vi "Create Analog Waveform.vi"(8 "error in (no error)":errorcluster, 9 "Type (0: awfSine)":i32(ring) items=["awfSine", "awfLoDistSine", "awfPhasedSine", "awfNoise", "awfUSASI", "awfSquare", "awfRamp", "awfArb", "awfChirp", "awfMultiTone", "awfIMD", "awfSyncBurstSine", "awfDC", "awfPolarity", "awfMLS", "awfLogSine"], 10 "Channel (0: A)":i32(ring) items=["A", "B"], 11 "VISA resource name":refnum<visa-resource-name>) -> (0 "error out":errorcluster, 2 "Waveform Channel ID":i32, 3 "VISA resource name out":refnum<visa-resource-name>)   [LabVIEW 2014, in "Stanford Research SR1.lvlib"]
doc: "Adds a waveform of the specified type to the generator channel and returns the ID of the newly created waveform."
uses:
  Stanford Research SR1.lvlib
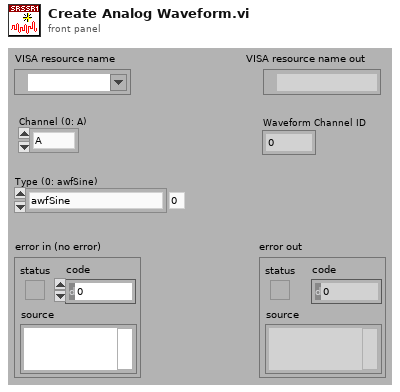
[diagram p1: front panel]
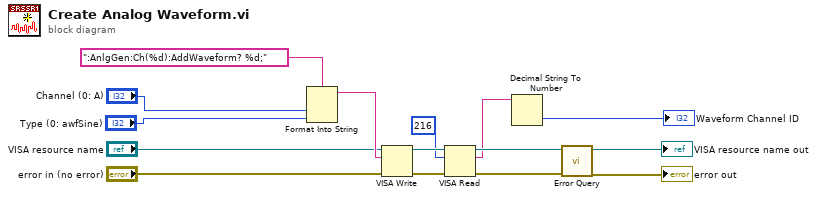
[diagram p0: block diagram]
diagram:
  n1 = Format Into String(format string=":AnlgGen:Ch(%d):AddWaveform? %d;", "Channel (0: A)", "Type (0: awfSine)") -> (resulting string=w15:string)  [unwired: 2 in, 1 out]
  n2 = VISA Write(VISA resource name="VISA resource name", write buffer=w15, error in (no error)="error in (no error)") -> (VISA resource name out=w8:refnum<visa-resource-name>, error out=w7:errorcluster)  [unwired: 1 out]
  n3 = VISA Read(VISA resource name=w8, byte count=u32 216, error in (no error)=w7) -> (VISA resource name out=w5:refnum<visa-resource-name>, read buffer=w2:string, error out=w4:errorcluster)  [unwired: 1 out]
  n4 = Decimal String To Number(string=w2) -> (number=→"Waveform Channel ID":i32)  [unwired: 2 in, 1 out]
  n5 = call "Error Query.vi"("error in (no error)"=w4, "VISA resource name"=w5) -> ("error out"=→"error out":errorcluster, "VISA resource name out"=→"VISA resource name out":refnum<visa-resource-name>)  [unwired: 6 in, 2 out]
